vi "Clear All.vi"(8 "error in (no error)":errorcluster, 11 "StorageService in":refnum<class "StorageService.lvclass">) -> (0 "error out":errorcluster, 3 "StorageService out":refnum<class "StorageService.lvclass">)   [LabVIEW 2014, in "StorageService.lvclass"]
uses:
  StorageService.lvclass
  StorageService.lvclass/StorageService.ctl
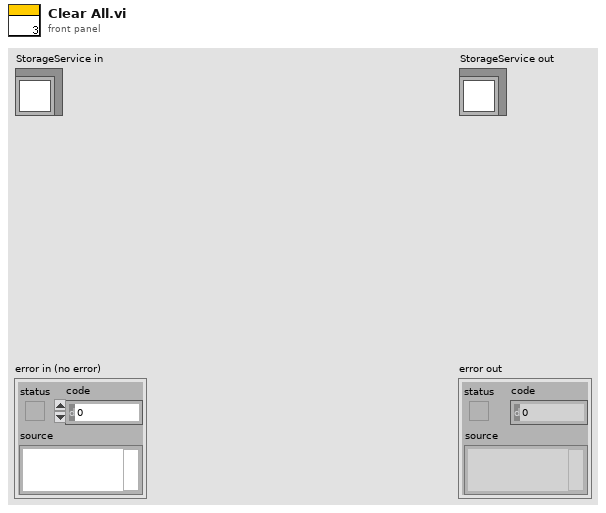
[diagram p1: front panel]
types:
  T1 = typedef "StorageService.lvclass/RegisteredObject.ctl" = cluster{"Name":string, "Is Acquired":bool, "Queue":refnum<queue>, "Message To Send":cluster{"Enqueuer":refnum<class "Message Enqueuer.lvclass">, "Message":refnum<class "ReplayData Msg.lvclass">}, "Save Parameters":variant}
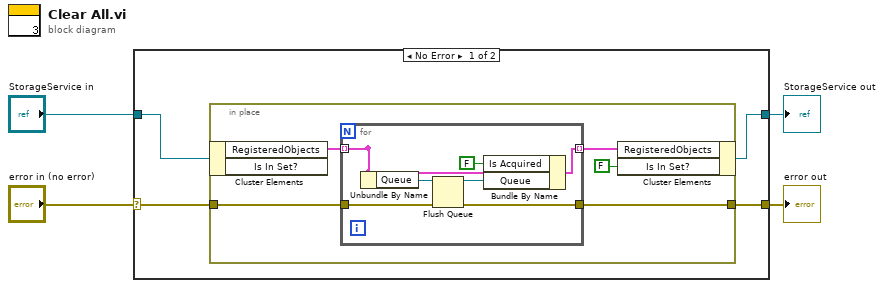
[diagram p0: block diagram]
diagram:
  n1 = case shown="No Error" "error in (no error)" {
    selector: "error in (no error)" -> [w6 w22]
    tunnel: [w5 w22] -> w3
    tunnel: [w7 w21] -> w1
    tunnel: "StorageService in" -> [w8 w21]
    frame No Error {
      n2 = in-place {
        in-place-border: w6 -> [w10]
        in-place-border: [w9] -> w5
        n3 = in-place-cluster #1(w8) -> ("RegisteredObjects"=w13:T1[])  [unwired: 1 out]
        n4 = for {
          tunnel: [w18] -> _ mode=indexing
          tunnel: w13 -> [w18] mode=indexing
          tunnel: [w17] -> w12 mode=indexing
          tunnel: w10 -> [w19]
          tunnel: [w14] -> w9
          n5 = Unbundle By Name(w18) -> ("Queue"=w20:refnum<queue>)
          n6 = Flush Queue(queue=w20, error in (no error)=w19) -> (queue out=w16:refnum<queue>, error out=w14:errorcluster)  [unwired: 1 out]
          n7 = Bundle By Name(cluster=w18, "Is Acquired"=FALSE, "Queue"=w16) -> (w17:T1)
        }
        n8 = in-place-cluster #1("RegisteredObjects"=w12, "Is In Set?"=FALSE) -> (w7:refnum<class "StorageService.lvclass">)
      }
    }
    frame Error {
    }
  }
  "error out" <- w3
  "StorageService out" <- w1
